vi "Channel_info_to_string.vi"(1 "Board type":T1=enum."NB-MIO-16H", 2 "ch info array":dbl[][](array[numeric]) format="%.2f", 3 "Ch & spans":T2[](array[typedef]) {"low limit (-10V)" format="%.3f"; "high limit (10V)" format="%.3f"}) -> (0 "Output string":string)   [LabVIEW 2010]
uses:
  Controls/Ch_and_Spans.ctl
  Controls/Board_Types.ctl
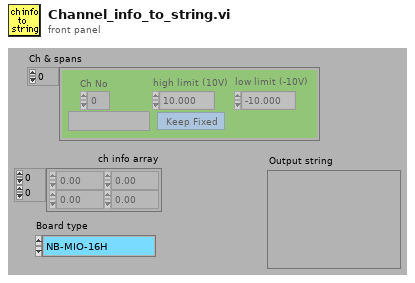
[diagram p1: front panel]
types:
  T1 = typedef "Board_Types.ctl" = enum16{"Simulate", "NB-MIO-16H", "PCI-MIO-16E", "6000E Series", "USB-92xx", "ADC488", "Lab-NB", "NB-DIO-24", "NI-DAQmx", "Local ADAM", "Server Channels"}
  T2 = typedef "Ch_and_Spans.ctl" = cluster{"high limit (10V)":sgl, "low limit (-10V)":sgl, "Ch No":i16, "Var name":string, "Use Latest Calib":bool}
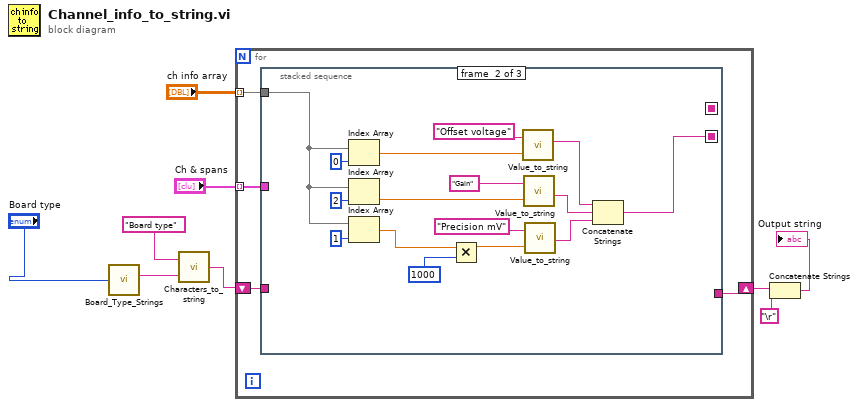
[diagram p0: block diagram]
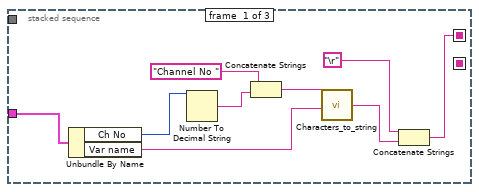
[diagram p2: hidden frame]
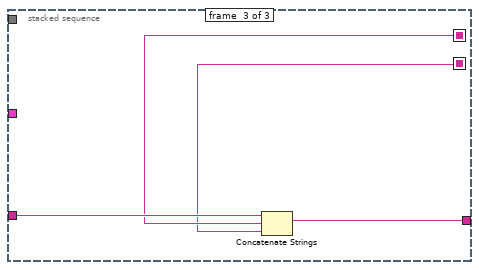
[diagram p3: hidden frame]
diagram:
  n1 = call "Board_Type_Strings.vi"("Board type"="Board type") -> ("Board String"=w2:string)  [unwired: 1 out]
  n2 = call "Characters_to_string.vi"("Characters to write"=w2, "Label for characters"="Board type") -> ("Output string"=w4:string)
  n3 = for {
    shift-right: [w11] -> w7
    shift-left: w4 -> [w12]
    tunnel: "Ch & spans" -> [w13] mode=indexing
    tunnel: "ch info array" -> [w10] mode=indexing
    n4 = stacked-sequence {
      seq-local: [w15 _ _] -> [_ _ w40]
      seq-local: [_ w23 _] -> [_ _ w39]
      tunnel: w13 -> [w22 _ _]
      tunnel: w12 -> [_ _ w42]
      tunnel: [_ _ w41] -> w11
      tunnel: w10 -> [_ w30 _]
      frame #0 {
        n5 = Unbundle By Name(w22) -> ("Ch No"=w20:i16, "Var name"=w17:string)
        n6 = Number To Decimal String(number=w20) -> (decimal integer string=w19:string)  [unwired: 1 in]
        n7 = Concatenate Strings("Channel No ", w19) -> (w18:string)
        n8 = call "Characters_to_string.vi"("Characters to write"=w17, "Label for characters"=w18) -> ("Output string"=w16:string)
        n9 = Concatenate Strings("\r", w16) -> (w15:string)
      }
      frame #1 {
        n10 = Index Array(array=w30, index=0) -> (element=w25:dbl)
        n11 = Index Array(array=w30, index=2) -> (element=w26:dbl)
        n12 = Index Array(array=w30, index=1) -> (element=w28:dbl)
        n13 = Multiply(x=w28, y=1000) -> (x*y=w27:dbl)
        n14 = call "Value_to_string.vi"("Value"=w25, "Label for value"="Offset voltage") -> ("Output string"=w24:string)  [unwired: 1 in]
        n15 = call "Value_to_string.vi"("Value"=w26, "Label for value"="Gain") -> ("Output string"=w38:string)  [unwired: 1 in]
        n16 = call "Value_to_string.vi"("Value"=w27, "Label for value"="Precision mV") -> ("Output string"=w37:string)  [unwired: 1 in]
        n17 = Concatenate Strings(w24, w38, w37) -> (w23:string)
      }
      frame #2 {
        n18 = Concatenate Strings(w42, w40, w39) -> (w41:string)
      }
    }
  }
  n19 = Concatenate Strings(w7, "\r") -> (→"Output string":string)
